vi "Loop Timer [Sequence].vi"() -> ()   [LabVIEW 2017]
panel:
  out "While Loop Time (ms)":u32
  out "For Loop Time (ms)":u32
  out "While Loop Array":i32[](array[numeric])
  out "For Loop Array":i32[](array[numeric])
  in  "Number of Elements":i32=10000000
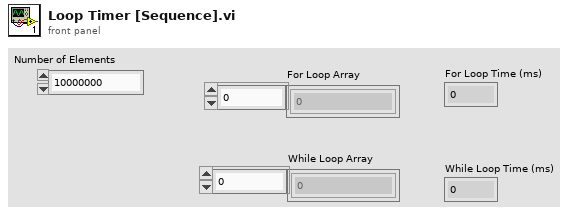
[diagram p1: front panel]
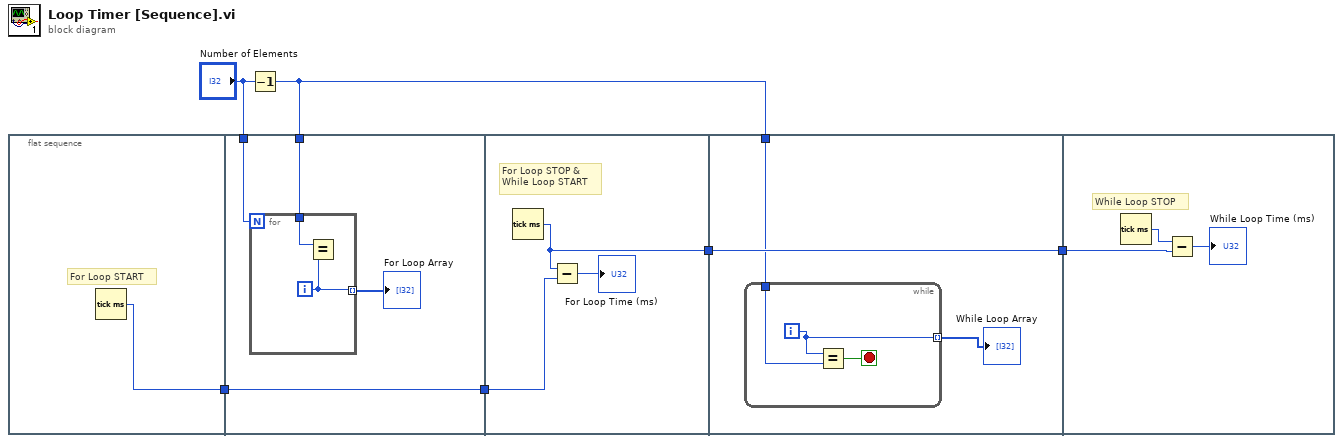
[diagram p0: block diagram]
diagram:
  n1 = flat-sequence {
    tunnel: [w7] -> w6
    tunnel: "Number of Elements" -> [w11]
    tunnel: w6 -> [w9]
    tunnel: [w9] -> w5
    tunnel: w1 -> [w8]
    tunnel: w5 -> [w16]
    tunnel: [w14] -> w3
    tunnel: [w19] -> w4
    tunnel: w3 -> [w19]
    tunnel: w1 -> [w18]
    tunnel: w4 -> [w24]
    frame #0 {
      # "For Loop START"
      n2 = Tick Count (ms)() -> (millisecond timer value=w7:u32)
    }
    frame #1 {
      n3 = for {
        N: w11 -> [_]
        tunnel: [w13] -> w10 mode=indexing
        tunnel: w8 -> [w12]
        i -> [w13]
        n4 = Equal?(x=w12, y=w13) -> ()  [unwired: 1 out]
      }
      "For Loop Array" <- w10
    }
    frame #2 {
      # "For Loop STOP &\nWhile Loop START"
      n5 = Tick Count (ms)() -> (millisecond timer value=w14:u32)
      n6 = Subtract(x=w14, y=w16) -> (x-y=→"For Loop Time (ms)":u32)
    }
    frame #3 {
      n7 = while {
        tunnel: w18 -> [w21]
        tunnel: [w20] -> w17 mode=indexing
        i -> [w20]
        stop <- w22 stop-if-true
        n8 = Equal?(x=w20, y=w21) -> (x = y?=w22:bool)
      }
      "While Loop Array" <- w17
    }
    frame #4 {
      # "While Loop STOP"
      n9 = Tick Count (ms)() -> (millisecond timer value=w25:u32)
      n10 = Subtract(x=w25, y=w24) -> (x-y=→"While Loop Time (ms)":u32)
    }
  }
  n11 = Decrement(x="Number of Elements") -> (x-1=w1:i32)
